vi "fileInfo.vi"(7 "LabVIEW Web Service Request":refnum<class "Web Request.lvclass">) -> ()   [LabVIEW 2014]
uses:
  <vilib>/wsapi/Web Request.lvclass
panel:
  out "resulting string":string
  # "Use the Web Service Request input terminal to call the VIs on the Web Services palette. Do not remove it from the connector pane unless you don't need access to the palette."
  # "Each additional control wired to the connector pane will be available as an input in the URL. To include an indicator in terminal-mode output (the default setting), it must also be wired to the connector pane."
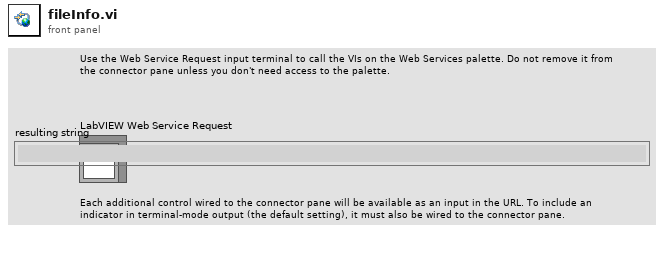
[diagram p1: front panel]
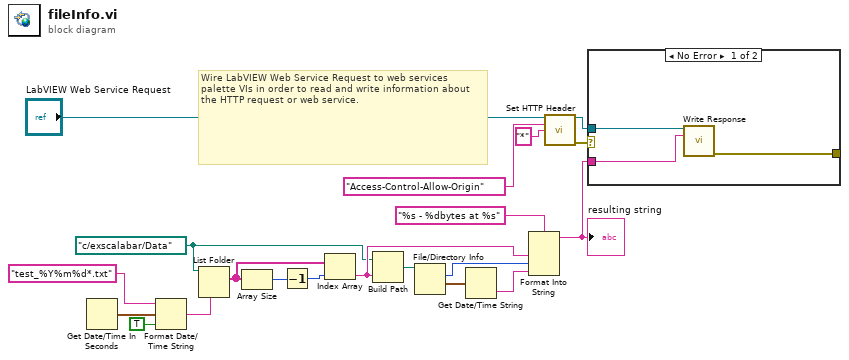
[diagram p0: block diagram]
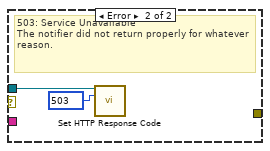
[diagram p2: hidden frame]
diagram:
  w14 = path "c:/exscalabar/Data" ("path")
  # "Wire LabVIEW Web Service Request to web services palette VIs in order to read and write information about the HTTP request or web service."
  n1 = Get Date/Time In Seconds() -> (seconds since 1Jan1904=w3:timestamp)
  n2 = Format Date/Time String(time format string (%c)="test_%Y%m%d*.txt", seconds (now)=w3, UTC format=TRUE) -> (date/time string=w1:string)
  n3 = List Folder(path=w14, pattern=w1) -> (filenames=w11:string[])  [unwired: 2 in, 3 out]
  n4 = Array Size(array=w11) -> (size(s)=w12:i32)
  n5 = Decrement(x=w12) -> (x-1=w13:i32)
  n6 = Index Array(array=w11, index=w13) -> (element=w17:string)
  n7 = Build Path(base path=w14, name or relative path=w17) -> (appended path=w15:path)
  n8 = File/Directory Info(path=w15) -> (size=w18:i64, last mod=w19:timestamp)  [unwired: 1 in, 5 out]
  n9 = Get Date/Time String(seconds (now)=w19) -> (time string=w20:string)  [unwired: 2 in, 1 out]
  n10 = Format Into String(format string="%s - %dbytes at %s", w17, w18, w20) -> (resulting string=w5:string)  [unwired: 2 in, 1 out]
  "resulting string" <- w5
  n11 = call <vilib>:"Set HTTP Header.vi"("LabVIEW Web Service Request"="LabVIEW Web Service Request", "header"="Access-Control-Allow-Origin", "header value"="*") -> ("LabVIEW Web Service Request out"=w6:refnum<class "Web Request.lvclass">, "error out"=w7:errorcluster)  [unwired: 11 in]
  n12 = case shown="No Error" w7 {
    tunnel: w6 -> [w23 w25]
    tunnel: w5 -> [w22 _]
    tunnel: [w21 _] -> _
    frame No Error {
      n13 = call <vilib>:"Write Response.vi"("LabVIEW Web Service Request"=w23, "response string"=w22) -> ("error out"=w21:errorcluster)  [unwired: 12 in, 1 out]
    }
    frame Error {
      w24 = 503 items=["100"=100, "101"=101, "200"=200, "201"=201, "202"=202, "203"=203, "204"=204, "205"=205, "206"=206, "300"=300, "301"=301, "302"=302, "303"=303, "304"=304, "305"=305, "306"=306, "307"=307, "400"=400, "401"=401, "402"=402, "403"=403, "404"=404, "405"=405, "406"=406, "407"=407, "408"=408, "409"=409, "410"=410, "411"=411, "412"=412, "413"=413, "414"=414, "415"=415, "416"=416, "417"=417, "500"=500, "501"=501, "502"=502, "503"=503, "504"=504, "505"=505] ("response code (200)")
      # "503: Service Unavailable\nThe notifier did not return properly for whatever reason."
      n14 = call <vilib>:"Set HTTP Response Code.vi"("LabVIEW Web Service Request"=w25, "response code (200)"=w24) -> ()  [unwired: 12 in, 2 out]
    }
  }
